vi "Digital_Bridge_3_kart.vi"() -> ()   [LabVIEW 2014] (continued)
                    n5059 = local write "IF ELSE Y 5"(w1698) -> ()
                    n5060 = local write "Y1 2"(w1698) -> ()
                    n5061 = local write "IF ELSE Y"(w1698) -> ()
                    n5062 = local write "X1 3"(w1698) -> ()
                    n5063 = local write "IF ELSE X"(w1698) -> ()
                    n5064 = local write "Y1 3"(w1698) -> ()
                    n5065 = local write "RANGE KONTROL X"(w1698) -> ()
                    n5066 = local write "Y 4"(w1698) -> ()
                    n5067 = local write "RANGE KONTROL Y 2"(w1698) -> ()
                    n5068 = local write "Y"(w1698) -> ()
                    n5069 = local write "RANGE KONTROL Y 3"(w1698) -> ()
                    n5070 = local write "X 5"(w1698) -> ()
                    n5071 = local write "RANGE KONTROL X 4"(w1698) -> ()
                    n5072 = local write "Y 5"(w1698) -> ()
                    n5073 = local write "RANGE KONTROL Y 4"(w1698) -> ()
                    n5074 = local write "IF ELSE Y 2"(w1698) -> ()
                    n5075 = local write "X1 4"(w1698) -> ()
                    n5076 = local write "IF ELSE X 2"(w1698) -> ()
                    n5077 = local write "Y1 4"(w1698) -> ()
                    n5078 = local write "IF ELSE Y 3"(w1698) -> ()
                    n5079 = local write "X1 5"(w1698) -> ()
                    n5080 = local write "IF ELSE X 3"(w1698) -> ()
                    n5081 = local write "Y1 5"(w1698) -> ()
                    n5082 = local write "IF ELSE X 4"(w1698) -> ()
                    "Boolean 5" <- w1696
                    "Boolean 3" <- w1696
                    "Boolean 2" <- w1696
                    "Boolean 4" <- w1696
                    "Boolean" <- w1696
                  }
                }
                n5083 = flat-sequence {
                  frame #0 {
                    w1411 = dbl[][] [] ("Other Array")
                    w1412 = dbl[][] [] ("Other Array")
                    "Denge Kosulu x2_y2" <- w1412
                    "Denge Kosulu x1_x2" <- w1412
                    "Denge Kosulu y1_y2" <- w1412
                    "Output Denge Kosulu x2_y2" <- w1411
                    "Output Denge Kosulu x1_x2" <- w1411
                    "Outpu Denge Kosulu y1_y2" <- w1411
                  }
                  frame #1 {
                    n5084 = Initialize Array(0.0 ("element"), 10 ("dimension size"), 20 ("dimension size")) -> (w1416:dbl[][])
                    n5085 = Initialize Array(0.0 ("element"), 10 ("dimension size"), 20 ("dimension size")) -> (w1417:dbl[][])
                    n5086 = Initialize Array(0.0 ("element"), 10 ("dimension size"), 20 ("dimension size")) -> (w1418:dbl[][])
                    n5087 = local write "Denge Kosulu x2_y2"(w1418) -> ()
                    n5088 = local write "Denge Kosulu y1_y2"(w1416) -> ()
                    n5089 = local write "Denge Kosulu x1_x2"(w1417) -> ()
                  }
                  frame #2 {
                    n5090 = for {
                      N: 20 -> [_]
                      i -> [w1426]
                      n5091 = for {
                        N: 10 -> [_]
                        tunnel: w1426 -> [w1428]
                        i -> [w1431]
                        n5092 = local read "Denge Kosulu x2_y2"() -> (w1430:dbl[][])
                        n5093 = case shown="5" w1431 {
                          tunnel: w1431 -> [w1435 w1439 w1445 w1450 w1455 w1460 w1465 w1470 w1475 w1480]
                          tunnel: w1430 -> [w1434 w1438 w1444 w1449 w1454 w1459 w1464 w1469 w1474 w1479]
                          tunnel: [w1433 w1440 w1443 w1448 w1453 w1458 w1463 w1468 w1473 w1478] -> w1429
                          tunnel: w1428 -> [w1432 w1437 w1442 w1447 w1452 w1457 w1462 w1467 w1472 w1477]
                          frame 0, Default {
                            n5094 = local read "AD X_2"() -> (w1436:dbl)
                            n5095 = Replace Array Subset(array=w1434, new element=w1436, index (row)=w1435, index (col)=w1432) -> (w1433:dbl[][])
                          }
                          frame 1 {
                            n5096 = local read "AD Y_2"() -> (w1441:dbl)
                            n5097 = Replace Array Subset(array=w1438, new element=w1441, index (row)=w1439, index (col)=w1437) -> (w1440:dbl[][])
                          }
                          frame 2 {
                            n5098 = local read "10R X_2"() -> (w1446:dbl)
                            n5099 = Replace Array Subset(array=w1444, new element=w1446, index (row)=w1445, index (col)=w1442) -> (w1443:dbl[][])
                          }
                          frame 3 {
                            n5100 = local read "10R Y_2"() -> (w1451:dbl)
                            n5101 = Replace Array Subset(array=w1449, new element=w1451, index (row)=w1450, index (col)=w1447) -> (w1448:dbl[][])
                          }
                          frame 4 {
                            n5102 = local read "1R X_2"() -> (w1456:dbl)
                            n5103 = Replace Array Subset(array=w1454, new element=w1456, index (row)=w1455, index (col)=w1452) -> (w1453:dbl[][])
                          }
                          frame 5 {
                            n5104 = local read "1R Y_2"() -> (w1461:dbl)
                            n5105 = Replace Array Subset(array=w1459, new element=w1461, index (row)=w1460, index (col)=w1457) -> (w1458:dbl[][])
                          }
                          frame 6 {
                            n5106 = local read "Wagner X_2"() -> (w1466:dbl)
                            n5107 = Replace Array Subset(array=w1464, new element=w1466, index (row)=w1465, index (col)=w1462) -> (w1463:dbl[][])
                          }
                          frame 7 {
                            n5108 = local read "Wagner Y_2"() -> (w1471:dbl)
                            n5109 = Replace Array Subset(array=w1469, new element=w1471, index (row)=w1470, index (col)=w1467) -> (w1468:dbl[][])
                          }
                          frame 8 {
                            n5110 = local read "Kelvin X_2"() -> (w1476:dbl)
                            n5111 = Replace Array Subset(array=w1474, new element=w1476, index (row)=w1475, index (col)=w1472) -> (w1473:dbl[][])
                          }
                          frame 9 {
                            n5112 = local read "Kelvin Y_2"() -> (w1481:dbl)
                            n5113 = Replace Array Subset(array=w1479, new element=w1481, index (row)=w1480, index (col)=w1477) -> (w1478:dbl[][])
                          }
                        }
                        n5114 = local write "Denge Kosulu x2_y2"(w1429) -> ()
                      }
                    }
                  }
                  frame #3 {
                    n5115 = for {
                      N: 20 -> [_]
                      i -> [w1483]
                      n5116 = for {
                        N: 10 -> [_]
                        tunnel: w1483 -> [w1485]
                        i -> [w1488]
                        n5117 = local read "Denge Kosulu x1_x2"() -> (w1487:dbl[][])
                        n5118 = case shown="0, Default" w1488 {
                          tunnel: w1488 -> [w1492 w1496 w1502 w1507 w1512 w1517 w1522 w1527 w1532 w1537]
                          tunnel: w1487 -> [w1491 w1495 w1501 w1506 w1511 w1516 w1521 w1526 w1531 w1536]
                          tunnel: [w1490 w1497 w1500 w1505 w1510 w1515 w1520 w1525 w1530 w1535] -> w1486
                          tunnel: w1485 -> [w1489 w1494 w1499 w1504 w1509 w1514 w1519 w1524 w1529 w1534]
                          frame 0, Default {
                            n5119 = local read "AD X_1"() -> (w1493:dbl)
                            n5120 = Replace Array Subset(array=w1491, new element=w1493, index (row)=w1492, index (col)=w1489) -> (w1490:dbl[][])
                          }
                          frame 1 {
                            n5121 = local read "AD X_2"() -> (w1498:dbl)
                            n5122 = Replace Array Subset(array=w1495, new element=w1498, index (row)=w1496, index (col)=w1494) -> (w1497:dbl[][])
                          }
                          frame 2 {
                            n5123 = local read "10R X_1"() -> (w1503:dbl)
                            n5124 = Replace Array Subset(array=w1501, new element=w1503, index (row)=w1502, index (col)=w1499) -> (w1500:dbl[][])
                          }
                          frame 3 {
                            n5125 = local read "10R X_2"() -> (w1508:dbl)
                            n5126 = Replace Array Subset(array=w1506, new element=w1508, index (row)=w1507, index (col)=w1504) -> (w1505:dbl[][])
                          }
                          frame 4 {
                            n5127 = local read "1R X_1"() -> (w1513:dbl)
                            n5128 = Replace Array Subset(array=w1511, new element=w1513, index (row)=w1512, index (col)=w1509) -> (w1510:dbl[][])
                          }
                          frame 5 {
                            n5129 = local read "1R X_2"() -> (w1518:dbl)
                            n5130 = Replace Array Subset(array=w1516, new element=w1518, index (row)=w1517, index (col)=w1514) -> (w1515:dbl[][])
                          }
                          frame 6 {
                            n5131 = local read "Wagner X_1"() -> (w1523:dbl)
                            n5132 = Replace Array Subset(array=w1521, new element=w1523, index (row)=w1522, index (col)=w1519) -> (w1520:dbl[][])
                          }
                          frame 7 {
                            n5133 = local read "Wagner X_2"() -> (w1528:dbl)
                            n5134 = Replace Array Subset(array=w1526, new element=w1528, index (row)=w1527, index (col)=w1524) -> (w1525:dbl[][])
                          }
                          frame 8 {
                            n5135 = local read "Kelvin X_1"() -> (w1533:dbl)
                            n5136 = Replace Array Subset(array=w1531, new element=w1533, index (row)=w1532, index (col)=w1529) -> (w1530:dbl[][])
                          }
                          frame 9 {
                            n5137 = local read "Kelvin X_2"() -> (w1538:dbl)
                            n5138 = Replace Array Subset(array=w1536, new element=w1538, index (row)=w1537, index (col)=w1534) -> (w1535:dbl[][])
                          }
                        }
                        n5139 = local write "Denge Kosulu x1_x2"(w1486) -> ()
                      }
                    }
                  }
                  frame #4 {
                    n5140 = for {
                      N: 20 -> [_]
                      i -> [w1540]
                      n5141 = for {
                        N: 10 -> [_]
                        tunnel: w1540 -> [w1542]
                        i -> [w1545]
                        n5142 = local read "Denge Kosulu y1_y2"() -> (w1544:dbl[][])
                        n5143 = case shown="8" w1545 {
                          tunnel: w1545 -> [w1549 w1553 w1559 w1564 w1569 w1574 w1579 w1584 w1589 w1594]
                          tunnel: w1544 -> [w1548 w1552 w1558 w1563 w1568 w1573 w1578 w1583 w1588 w1593]
                          tunnel: [w1547 w1554 w1557 w1562 w1567 w1572 w1577 w1582 w1587 w1592] -> w1543
                          tunnel: w1542 -> [w1546 w1551 w1556 w1561 w1566 w1571 w1576 w1581 w1586 w1591]
                          frame 0, Default {
                            n5144 = local read "AD Y_1"() -> (w1550:dbl)
                            n5145 = Replace Array Subset(array=w1548, new element=w1550, index (row)=w1549, index (col)=w1546) -> (w1547:dbl[][])
                          }
                          frame 1 {
                            n5146 = local read "AD Y_2"() -> (w1555:dbl)
                            n5147 = Replace Array Subset(array=w1552, new element=w1555, index (row)=w1553, index (col)=w1551) -> (w1554:dbl[][])
                          }
                          frame 2 {
                            n5148 = local read "10R  Y_1"() -> (w1560:dbl)
                            n5149 = Replace Array Subset(array=w1558, new element=w1560, index (row)=w1559, index (col)=w1556) -> (w1557:dbl[][])
                          }
                          frame 3 {
                            n5150 = local read "10R Y_2"() -> (w1565:dbl)
                            n5151 = Replace Array Subset(array=w1563, new element=w1565, index (row)=w1564, index (col)=w1561) -> (w1562:dbl[][])
                          }
                          frame 4 {
                            n5152 = local read "1R Y_1"() -> (w1570:dbl)
                            n5153 = Replace Array Subset(array=w1568, new element=w1570, index (row)=w1569, index (col)=w1566) -> (w1567:dbl[][])
                          }
                          frame 5 {
                            n5154 = local read "1R Y_2"() -> (w1575:dbl)
                            n5155 = Replace Array Subset(array=w1573, new element=w1575, index (row)=w1574, index (col)=w1571) -> (w1572:dbl[][])
                          }
                          frame 6 {
                            n5156 = local read "Wagner Y_1"() -> (w1580:dbl)
                            n5157 = Replace Array Subset(array=w1578, new element=w1580, index (row)=w1579, index (col)=w1576) -> (w1577:dbl[][])
                          }
                          frame 7 {
                            n5158 = local read "Wagner Y_2"() -> (w1585:dbl)
                            n5159 = Replace Array Subset(array=w1583, new element=w1585, index (row)=w1584, index (col)=w1581) -> (w1582:dbl[][])
                          }
                          frame 8 {
                            n5160 = local read "Kelvin Y_1"() -> (w1590:dbl)
                            n5161 = Replace Array Subset(array=w1588, new element=w1590, index (row)=w1589, index (col)=w1586) -> (w1587:dbl[][])
                          }
                          frame 9 {
                            n5162 = local read "Kelvin Y_2"() -> (w1595:dbl)
                            n5163 = Replace Array Subset(array=w1593, new element=w1595, index (row)=w1594, index (col)=w1591) -> (w1592:dbl[][])
                          }
                        }
                        n5164 = local write "Denge Kosulu y1_y2"(w1543) -> ()
                      }
                    }
                  }
                }
                n5165 = flat-sequence {
                  frame #0 {
                    w1607 = 0.0 ("result output x [Wagner]")
                    w1609 = 0.0 ("output 2 y [10R]")
                    w1610 = 0.0 ("input 2 x [kelvin]")
                    w1611 = 0.0 ("input 1 x [kelvin]")
                    w1614 = 0.0 ("iterasyon ana denge")
                    w1615 = 0.0 ("iterasyon ana denge")
                    w1613 = 0.0 ("input 1 x [10R]")
                    w1612 = 0.0 ("iterasyon ana denge")
                    n5166 = global read "First_input_values.vi" "Active"() -> (w1606:bool)
                    n5167 = case shown="True" w1606 {
                      frame False {
                        n5168 = global read "First_input_values.vi" "Y 2. input 1R"() -> (→"Y 2.input 1R" →"1R Y(k-1)":dbl)
                        n5169 = global read "First_input_values.vi" "Y 1. input 1R"() -> (→"Y 1.input 1R" →"1R Yk":dbl)
                        n5170 = global read "First_input_values.vi" "X 2. input 1R"() -> (→"X 2.input 1R" →"1R X(k-1)":dbl)
                        n5171 = global read "First_input_values.vi" "X 1. input 1R"() -> (→"X 1.input 1R" →"1R Xk":dbl)
                        n5172 = global read "First_input_values.vi" "X 1. input 10R"() -> (→"X 1.input 10R" →"10R Xk":dbl)
                        n5173 = global read "First_input_values.vi" "X 2. input 10R"() -> (→"X 2.input 10R" →"10R X(k-1)":dbl)
                        n5174 = global read "First_input_values.vi" "X 1. input AD"() -> (→"X 1.input AD" →"AD Xk":dbl)
                        n5175 = global read "First_input_values.vi" "X 2. input AD"() -> (→"X 2.input AD" →"AD X(k-1)":dbl)
                        n5176 = global read "First_input_values.vi" "Y 2. input AD"() -> (→"Y 2.input AD" →"AD Y(k-1)":dbl)
                        n5177 = global read "First_input_values.vi" "Y 2. input 10R"() -> (→"Y 2.input 10R" →"10R Y(k-1)":dbl)
                        n5178 = global read "First_input_values.vi" "Y 1. input AD"() -> (→"Y 1.input AD" →"AD Yk":dbl)
                        n5179 = global read "First_input_values.vi" "Y 1. input 10R"() -> (→"Y 1.input 10R" →"10R Yk":dbl)
                        n5180 = global read "First_input_values.vi" "Y 1. input KV"() -> (→"Y 1.input KV" →"Kelvin Yk":dbl)
                        n5181 = global read "First_input_values.vi" "Y 2. input KV"() -> (→"Y 2.input KV" →"Kelvin Y(k-1)":dbl)
                        n5182 = global read "First_input_values.vi" "X 1. input KV"() -> (→"X 1.input KV" →"Kelvin Xk":dbl)
                        n5183 = global read "First_input_values.vi" "X 2. input KV"() -> (→"X 2.input KV" →"Kelvin X(k-1)":dbl)
                        n5184 = global read "First_input_values.vi" "X 2. input W"() -> (→"X 2.input W" →"Wagner  X(k-1)":dbl)
                        n5185 = global read "First_input_values.vi" "X 1. input W"() -> (→"X 1.input W" →"Wagner Xk":dbl)
                        n5186 = global read "First_input_values.vi" "Y 1. input W"() -> (→"Y 1.input W" →"Wagner Yk":dbl)
                        n5187 = global read "First_input_values.vi" "Y 2. input W"() -> (→"Y 2.input W" →"Wagner Y(k-1)":dbl)
                        n5188 = global read "First_input_values.vi" "X range 10R"() -> (→"X Range 10R":dbl)
                        n5189 = global read "First_input_values.vi" "X range AD"() -> (→"X Range AD":dbl)
                        n5190 = global read "First_input_values.vi" "X range KV"() -> (→"X Range KV":dbl)
                        n5191 = global read "First_input_values.vi" "X range 1R"() -> (→"X Range 1R":dbl)
                        n5192 = global read "First_input_values.vi" "X range W"() -> (→"X Range W":dbl)
                        n5193 = global read "First_input_values.vi" "Y range 10R"() -> (→"Y Range 10R":dbl)
                        n5194 = global read "First_input_values.vi" "Y range AD"() -> (→"Y Range AD":dbl)
                        n5195 = global read "First_input_values.vi" "Y range KV"() -> (→"Y Range KV":dbl)
                        n5196 = global read "First_input_values.vi" "Y range 1R"() -> (→"Y Range 1R":dbl)
                        n5197 = global read "First_input_values.vi" "Y range W"() -> (→"Y Range W":dbl)
                      }
                      frame True {
                        n5198 = for {
                          N: 6 -> [_]
                          i -> [w1648]
                          n5199 = for {
                            N: 5 -> [_]
                            tunnel: w1648 -> [w1651]
                            i -> [w1650]
                            n5200 = global read "First_input_values.vi" "Multi Values"() -> (w1653:dbl[][][])
                            n5201 = Index Array(array=w1653, index (dim 0)=0 ("index (page)"), index (dim 1)=w1651, index (dim 2)=w1650) -> (element=w1649:dbl)
                            n5202 = case shown="0, Default" w1651 {
                              tunnel: w1650 -> [w1655 w1662 w1669 w1676 w1683 w1690]
                              tunnel: w1649 -> [w1654 w1661 w1668 w1675 w1682 w1689]
                              frame 0, Default {
                                n5203 = case shown="0, Default" w1655 {
                                tunnel: w1654 -> [w1656 w1657 w1658 w1659 w1660]
                                frame 0, Default {
                                n5204 = local write "AD Xk"(w1656) -> ()
                                n5205 = local write "X 1.input AD"(w1656) -> ()
                                }
                                frame 1 {
                                n5206 = local write "10R Xk"(w1657) -> ()
                                n5207 = local write "X 1.input 10R"(w1657) -> ()
                                }
                                frame 2 {
                                n5208 = local write "1R Xk"(w1658) -> ()
                                n5209 = local write "X 1.input 1R"(w1658) -> ()
                                }
                                frame 3 {
                                n5210 = local write "Wagner Xk"(w1659) -> ()
                                n5211 = local write "X 1.input W"(w1659) -> ()
                                }
                                frame 4 {
                                n5212 = local write "Kelvin Xk"(w1660) -> ()
                                n5213 = local write "X 1.input KV"(w1660) -> ()
                                }
                                }
                              }
                              frame 1 {
                                n5214 = case shown="0, Default" w1662 {
                                tunnel: w1661 -> [w1663 w1664 w1665 w1666 w1667]
                                frame 0, Default {
                                n5215 = local write "AD X(k-1)"(w1663) -> ()
                                n5216 = local write "X 2.input AD"(w1663) -> ()
                                }
                                frame 1 {
                                n5217 = local write "10R X(k-1)"(w1664) -> ()
                                n5218 = local write "X 2.input 10R"(w1664) -> ()
                                }
                                frame 2 {
                                n5219 = local write "1R X(k-1)"(w1665) -> ()
                                n5220 = local write "X 2.input 1R"(w1665) -> ()
                                }
                                frame 3 {
                                n5221 = local write "Wagner  X(k-1)"(w1666) -> ()
                                n5222 = local write "X 2.input W"(w1666) -> ()
                                }
                                frame 4 {
                                n5223 = local write "Kelvin X(k-1)"(w1667) -> ()
                                n5224 = local write "X 2.input KV"(w1667) -> ()
                                }
                                }
                              }
                              frame 2 {
                                n5225 = case shown="2" w1669 {
                                tunnel: w1668 -> [w1670 w1671 w1672 w1673 w1674]
                                frame 0, Default {
                                n5226 = local write "X Range AD"(w1670) -> ()
                                }
                                frame 1 {
                                n5227 = local write "X Range 10R"(w1671) -> ()
                                }
                                frame 2 {
                                n5228 = local write "X Range 1R"(w1672) -> ()
                                }
                                frame 3 {
                                n5229 = local write "X Range W"(w1673) -> ()
                                }
                                frame 4 {
                                n5230 = local write "X Range KV"(w1674) -> ()
                                }
                                }
                              }
                              frame 3 {
                                n5231 = case shown="0, Default" w1676 {
                                tunnel: w1675 -> [w1677 w1678 w1679 w1680 w1681]
                                frame 0, Default {
                                n5232 = local write "AD Yk"(w1677) -> ()
                                n5233 = local write "Y 1.input AD"(w1677) -> ()
                                }
                                frame 1 {
                                n5234 = local write "10R Yk"(w1678) -> ()
                                n5235 = local write "Y 1.input 10R"(w1678) -> ()
                                }
                                frame 2 {
                                n5236 = local write "1R Yk"(w1679) -> ()
                                n5237 = local write "Y 1.input 1R"(w1679) -> ()
                                }
                                frame 3 {
                                n5238 = local write "Wagner Yk"(w1680) -> ()
                                n5239 = local write "Y 1.input W"(w1680) -> ()
                                }
                                frame 4 {
                                n5240 = local write "Kelvin Yk"(w1681) -> ()
                                n5241 = local write "Y 1.input KV"(w1681) -> ()
                                }
                                }
                              }
                              frame 4 {
                                n5242 = case shown="0, Default" w1683 {
                                tunnel: w1682 -> [w1684 w1685 w1686 w1687 w1688]
                                frame 0, Default {
                                n5243 = local write "AD Y(k-1)"(w1684) -> ()
                                n5244 = local write "Y 2.input AD"(w1684) -> ()
                                }
                                frame 1 {
                                n5245 = local write "10R Y(k-1)"(w1685) -> ()
                                n5246 = local write "Y 2.input 10R"(w1685) -> ()
                                }
                                frame 2 {
                                n5247 = local write "1R Y(k-1)"(w1686) -> ()
                                n5248 = local write "Y 2.input 1R"(w1686) -> ()
                                }
                                frame 3 {
                                n5249 = local write "Wagner Y(k-1)"(w1687) -> ()
                                n5250 = local write "Y 2.input W"(w1687) -> ()
                                }
                                frame 4 {
                                n5251 = local write "Kelvin Y(k-1)"(w1688) -> ()
                                n5252 = local write "Y 2.input KV"(w1688) -> ()
                                }
                                }
                              }
                              frame 5 {
                                n5253 = case shown="0, Default" w1690 {
                                tunnel: w1689 -> [w1691 w1692 w1693 w1694 w1695]
                                frame 0, Default {
                                n5254 = local write "Y Range AD"(w1691) -> ()
                                }
                                frame 1 {
                                n5255 = local write "Y Range 10R"(w1692) -> ()
                                }
                                frame 2 {
                                n5256 = local write "Y Range 1R"(w1693) -> ()
                                }
                                frame 3 {
                                n5257 = local write "Y Range W"(w1694) -> ()
                                }
                                frame 4 {
                                n5258 = local write "Y Range KV"(w1695) -> ()
                                }
                                }
                              }
                            }
                          }
                        }
                      }
                    }
                    "input 1 x [kelvin]" <- w1610
                    "input 2 x [kelvin]" <- w1610
                    "output 2 x [kelvin]" <- w1610
                    "output 1 x [kelvin]" <- w1610
                    "input 1 y [kelvin]" <- w1610
                    "input 2 y [kelvin]" <- w1610
                    "output 1 y [kelvin]" <- w1610
                    "output 2 y [kelvin]" <- w1610
                    "input 1 x [wagner]" <- w1611
                    "input 2 x [wagner]" <- w1611
                    "output 1 x [wagner]" <- w1611
                    "output 2 x [wagner]" <- w1611
                    "input 1 y [wagner]" <- w1611
                    "input 2 y [wagner]" <- w1611
                    "output 1 y [wagner]" <- w1611
                    "output 2 y [wagner]" <- w1611
                    "output 2 x [1R]" <- w1612
                    "output 1 x [1R]" <- w1612
                    "input 1 x [1R]" <- w1612
                    "input 2 x [1R]" <- w1612
                    "input 1 y [1R]" <- w1612
                    "input 2 y [1R]" <- w1612
                    "output 1 y [1R]" <- w1612
                    "output 2 y [1R]" <- w1612
                    "output 1 x [10R]" <- w1609
                    "input 1 x [10R]" <- w1609
                    "output 2 x [10R]" <- w1609
                    "input 2 x [10R]" <- w1609
                    "input 2 y [10R]" <- w1609
                    "output 2 y [10R]" <- w1609
                    "input 1 y [10R]" <- w1609
                    "output 1 y [10R]" <- w1609
                    "output 2 x [ana denge]" <- w1613
                    "output 1 x [ana denge]" <- w1613
                    "input 1 x [ana denge]" <- w1613
                    "input 2 x [ana denge]" <- w1613
                    "input 1 y [ana denge]" <- w1613
                    "input 2 y [ana denge]" <- w1613
                    "output 2 y [ana denge]" <- w1613
                    "output 1 y [ana denge]" <- w1613
                    "iterasyon KELVIN" <- w1615
                    "iterasyon WAGNER" <- w1615
                    "iterasyon 1R" <- w1615
                    "iterasyon 10R" <- w1615
                    "iterasyon AD" <- w1615
                    "İterasyon X" <- w1614
                    "İterasyon Y" <- w1614
                    "İterasyon X 2" <- w1614
                    "İterasyon Y 2" <- w1614
                    "İterasyon X 3" <- w1614
                    "İterasyon Y 3" <- w1614
                    "İterasyon X 4" <- w1614
                    "İterasyon Y 4" <- w1614
                    "İterasyon X 5" <- w1614
                    "İterasyon Y 5" <- w1614
                    "Iterasyon Successful" <- 0.0 ("Iterasyon Successful")
                    "result output x [Wagner]" <- w1607
                    "result output y [Wagner]" <- w1607
                    "result output x [1R]" <- w1607
                    "result output y [1R]" <- w1607
                    "result output x [10R]" <- w1607
                    "result output y [10R]" <- w1607
                    "result output x [AD]" <- w1607
                    "result output y [AD]" <- w1607
                    "result output x [Kelvin]" <- w1607
                    "result output y [Kelvin]" <- w1607
                  }
                }
                n5259 = flat-sequence {
                  frame #0 {
                    "Hatalar" <- string[] [] ("Hatalar")
                    "Frekanslar" <- i32[] []
                    "extra default values" <- i32[][] []
                    "control hz array" <- i32[][] []
                  }
                }
                n5260 = flat-sequence {
                  tunnel: [w1596] -> w1410
                  tunnel: w1410 -> [w1598]
                  frame #0 {
                    n5261 = property on="Frekans Listbox" class="LstBox (strict)"() -> ("Item Names"=w1596:string[])  [unwired: 2 in, 2 out]
                    n5262 = property on="Multicolumn Listbox" class="MCListbox (strict)"("RowHdrs[]"=w1596) -> ()  [unwired: 2 in, 2 out]
                  }
                  frame #1 {
                    n5263 = Array Size(array=w1598) -> (size(s)=w1597:i32)
                    n5264 = property on="Multicolumn Listbox" class="MCListbox (strict)"("NumRows"=w1597) -> ()  [unwired: 2 in, 2 out]
                  }
                  frame #2 {
                    n5265 = property on="Frekans Listbox" class="LstBox (strict)"() -> ("Item Names"=w1599:string[])  [unwired: 2 in, 2 out]
                    n5266 = Array Size(array=w1599) -> (size(s)=w1600:i32)
                    n5267 = for {
                      N: w1600 -> [_]
                      i -> [w1604]
                      n5268 = property on="Multicolumn Listbox" class="MCListbox (strict)"() -> ("RowHdrs[]"=w1602:string[])  [unwired: 2 in, 2 out]
                      n5269 = property on="Frekans Listbox" class="LstBox (strict)"() -> ("Item Names"=w1605:string[])  [unwired: 2 in, 2 out]
                      n5270 = Index Array(array=w1605, index=w1604) -> (element=w1603:string)
                      n5271 = Replace Array Subset(array=w1602, new element=w1603, index=w1604) -> (w1601:string[])
                      n5272 = property on="Multicolumn Listbox" class="MCListbox (strict)"("RowHdrs[]"=w1601) -> ()  [unwired: 2 in, 2 out]
                    }
                  }
                }
              }
              frame #1 {
                n5273 = local write "first process"(FALSE ("first process")) -> ()
              }
            }
          }
        }
        n5274 = case shown="True" "error" {
          frame False {
          }
          frame True {
            n5275 = disable-structure shown="Disabled" {
              frame Disabled {
                n5276 = local read "Denge Seçimi"() -> (w1765:u8)
                n5277 = Number To Fractional String(number=w1765) -> ()  [unwired: 3 in, 1 out]
              }
              frame Enabled {
              }
            }
            n5278 = local read "frekans index"() -> (w1762:dbl)
            n5279 = local read "Frekanslar"() -> (w1763:dbl[])
            n5280 = Index Array(array=w1763, index=w1762) -> (element=w1764:dbl)
            n5281 = Number To Decimal String(number=w1764) -> (decimal integer string=w1759:string)  [unwired: 1 in]
            n5282 = Concatenate Strings(w1759, " Hz dengelenemedi") -> (w1757:string)
            n5283 = flat-sequence {
              tunnel: [w1766] -> w1761
              tunnel: w1757 -> [w1766]
              tunnel: [w1768] -> w1760
              tunnel: w1761 -> [w1768]
              tunnel: w1760 -> [w1770]
              frame #0 {
                n5284 = Wait (ms)(milliseconds to wait=u32 1000) -> ()  [unwired: 1 out]
              }
              frame #1 {
                n5285 = disable-structure shown="Disabled" {
                  frame Disabled {
                    w1769 = "a" ("button name (\"OK\")")
                    n5286 = One Button Dialog(message=w1769, button name ("OK")=w1769) -> ()  [unwired: 1 out]
                  }
                  frame Enabled {
                  }
                }
              }
              frame #2 {
                n5287 = flat-sequence {
                  tunnel: w1770 -> [w1776]
                  tunnel: [w1774] -> w1773
                  tunnel: [w1777] -> w1772
                  tunnel: w1773 -> [w1777]
                  tunnel: [w1779] -> w1771
                  tunnel: w1772 -> [w1779]
                  tunnel: w1771 -> [w1781]
                  frame #0 {
                    n5288 = local read "Hatalar"() -> (w1775:string[])
                    n5289 = Build Array (concatenate)(w1776, w1775) -> (w1774:string[])
                  }
                  frame #1 {
                    n5290 = local write "Hatalar"(string[] [] ("Hatalar")) -> ()
                  }
                  frame #2 {
                    n5291 = Wait (ms)(milliseconds to wait=u32 100) -> ()  [unwired: 1 out]
                  }
                  frame #3 {
                    n5292 = local write "Hatalar"(w1781) -> ()
                  }
                }
              }
              frame #3 {
                n5293 = local write "reset values"(TRUE ("reset values")) -> ()
                n5294 = local write "error 2"(TRUE ("reset values")) -> ()
                n5295 = local write "error"(FALSE ("reset values")) -> ()
              }
            }
            n5296 = local read "input values"() -> (→"input values 2":dbl[])
          }
        }
        n5297 = case shown="True" "Wagner" {
          frame False {
          }
          frame True {
            n5298 = flat-sequence {
              frame #0 {
                w674 = u16 0 items=["Wagner", "Ground"] ("Switch")
                w673 = u16 1 items=["Open All", "Ana Denge", "10R", "1R"] ("Ring")
                n5299 = call "mux1.vi"("Ring"=w673) -> ("error out"=w672:errorcluster)  [unwired: 9 in]
                n5300 = call "mux2.vi"("Switch"=w674, "error in (no error)"=w672) -> ()  [unwired: 6 in, 1 out]
              }
              frame #1 {
                n5301 = Wait (ms)(milliseconds to wait=u32 100) -> ()  [unwired: 1 out]
              }
              frame #2 {
                w677 = u16 0 items=["A", "A-B"] ("Input Source (0: A)")
                n5302 = local read "GPIB In"() -> (w676:refnum<visa-resource-name>)
                n5303 = call "input source.vi"("Input Source (0: A)"=w677, "VISA resource name"=w676) -> ()  [unwired: 8 in, 2 out]
              }
              frame #3 {
                n5304 = Wait (ms)(milliseconds to wait=u32 100) -> ()  [unwired: 1 out]
              }
              frame #4 {
                n5305 = local write "Wagner"(FALSE) -> ()
              }
            }
          }
        }
        n5306 = case shown="True" "Kelvin" {
          frame False {
          }
          frame True {
            n5307 = flat-sequence {
              frame #0 {
                w666 = u16 1 items=["Wagner", "Ground"] ("Switch")
                w665 = u16 1 items=["Open All", "Ana Denge", "10R", "1R"] ("Ring")
                n5308 = call "mux1.vi"("Ring"=w665) -> ("error out"=w664:errorcluster)  [unwired: 9 in]
                n5309 = call "mux2.vi"("Switch"=w666, "error in (no error)"=w664) -> ()  [unwired: 6 in, 1 out]
              }
              frame #1 {
                n5310 = Wait (ms)(milliseconds to wait=u32 100) -> ()  [unwired: 1 out]
              }
              frame #2 {
                w669 = u16 1 items=["A", "A-B"] ("Input Source (0: A)")
                n5311 = local read "GPIB In"() -> (w668:refnum<visa-resource-name>)
                n5312 = call "input source.vi"("Input Source (0: A)"=w669, "VISA resource name"=w668) -> ()  [unwired: 8 in, 2 out]
              }
              frame #3 {
                n5313 = Wait (ms)(milliseconds to wait=u32 100) -> ()  [unwired: 1 out]
              }
              frame #4 {
                n5314 = local write "Kelvin"(FALSE) -> ()
              }
            }
          }
        }
        n5315 = case shown="True" "Open all" {
          frame False {
          }
          frame True {
            n5316 = flat-sequence {
              frame #0 {
                w658 = u16 1 items=["Wagner", "Ground"] ("Switch")
                w657 = u16 0 items=["Open All", "Ana Denge", "10R", "1R"] ("Ring")
                n5317 = call "mux1.vi"("Ring"=w657) -> ("error out"=w656:errorcluster)  [unwired: 9 in]
                n5318 = call "mux2.vi"("Switch"=w658, "error in (no error)"=w656) -> ()  [unwired: 6 in, 1 out]
              }
              frame #1 {
                n5319 = Wait (ms)(milliseconds to wait=u32 100) -> ()  [unwired: 1 out]
              }
              frame #2 {
                w661 = u16 0 items=["A", "A-B"] ("Input Source (0: A)")
                n5320 = local read "GPIB In"() -> (w660:refnum<visa-resource-name>)
                n5321 = call "input source.vi"("Input Source (0: A)"=w661, "VISA resource name"=w660) -> ()  [unwired: 8 in, 2 out]
              }
              frame #3 {
                n5322 = Wait (ms)(milliseconds to wait=u32 100) -> ()  [unwired: 1 out]
              }
              frame #4 {
                n5323 = local write "Open all"(FALSE) -> ()
              }
            }
          }
        }
        n5324 = case shown="True" "AD" {
          frame False {
          }
          frame True {
            n5325 = flat-sequence {
              frame #0 {
                w698 = u16 1 items=["Wagner", "Ground"] ("Switch")
                w697 = u16 1 items=["Open All", "Ana Denge", "10R", "1R"] ("Ring")
                n5326 = call "mux1.vi"("Ring"=w697) -> ("error out"=w696:errorcluster)  [unwired: 9 in]
                n5327 = call "mux2.vi"("Switch"=w698, "error in (no error)"=w696) -> ()  [unwired: 6 in, 1 out]
              }
              frame #1 {
                n5328 = Wait (ms)(milliseconds to wait=u32 100) -> ()  [unwired: 1 out]
              }
              frame #2 {
                w701 = u16 0 items=["A", "A-B"] ("Input Source (0: A)")
                n5329 = local read "GPIB In"() -> (w700:refnum<visa-resource-name>)
                n5330 = call "input source.vi"("Input Source (0: A)"=w701, "VISA resource name"=w700) -> ()  [unwired: 8 in, 2 out]
              }
              frame #3 {
                n5331 = Wait (ms)(milliseconds to wait=u32 100) -> ()  [unwired: 1 out]
              }
              frame #4 {
                n5332 = local write "AD"(FALSE) -> ()
              }
            }
          }
        }
        n5333 = case shown="True" "1R" {
          frame False {
          }
          frame True {
            n5334 = flat-sequence {
              frame #0 {
                w682 = u16 1 items=["Wagner", "Ground"] ("Switch")
                w681 = u16 3 items=["Open All", "Ana Denge", "10R", "1R"] ("Ring")
                n5335 = call "mux1.vi"("Ring"=w681) -> ("error out"=w680:errorcluster)  [unwired: 9 in]
                n5336 = call "mux2.vi"("Switch"=w682, "error in (no error)"=w680) -> ()  [unwired: 6 in, 1 out]
              }
              frame #1 {
                n5337 = Wait (ms)(milliseconds to wait=u32 100) -> ()  [unwired: 1 out]
              }
              frame #2 {
                w685 = u16 0 items=["A", "A-B"] ("Input Source (0: A)")
                n5338 = local read "GPIB In"() -> (w684:refnum<visa-resource-name>)
                n5339 = call "input source.vi"("Input Source (0: A)"=w685, "VISA resource name"=w684) -> ()  [unwired: 8 in, 2 out]
              }
              frame #3 {
                n5340 = Wait (ms)(milliseconds to wait=u32 100) -> ()  [unwired: 1 out]
              }
              frame #4 {
                n5341 = local write "1R"(FALSE) -> ()
              }
            }
          }
        }
        n5342 = case shown="True" "10R" {
          frame False {
          }
          frame True {
            n5343 = flat-sequence {
              frame #0 {
                w690 = u16 1 items=["Wagner", "Ground"] ("Switch")
                w689 = u16 2 items=["Open All", "Ana Denge", "10R", "1R"] ("Ring")
                n5344 = call "mux1.vi"("Ring"=w689) -> ("error out"=w688:errorcluster)  [unwired: 9 in]
                n5345 = call "mux2.vi"("Switch"=w690, "error in (no error)"=w688) -> ()  [unwired: 6 in, 1 out]
              }
              frame #1 {
                n5346 = Wait (ms)(milliseconds to wait=u32 100) -> ()  [unwired: 1 out]
              }
              frame #2 {
                w693 = u16 0 items=["A", "A-B"] ("Input Source (0: A)")
                n5347 = local read "GPIB In"() -> (w692:refnum<visa-resource-name>)
                n5348 = call "input source.vi"("Input Source (0: A)"=w693, "VISA resource name"=w692) -> ()  [unwired: 8 in, 2 out]
              }
              frame #3 {
                n5349 = Wait (ms)(milliseconds to wait=u32 100) -> ()  [unwired: 1 out]
              }
              frame #4 {
                n5350 = local write "10R"(FALSE) -> ()
              }
            }
          }
        }
        n5351 = call "Role_Auto_Secim.vi"("Activate"="Activate", "Denge Kolu"="Denge Kolu") -> ()  [unwired: 10 in]
        n5352 = case shown="True" "REFERANS FAZ" {
          frame False {
          }
          frame True {
            n5353 = flat-sequence {
              frame #0 {
                n5354 = local read "GPIB In"() -> (w4267:refnum<visa-resource-name>)
                n5355 = call "reference phase.vi"("Reference Phase (0.000 degrees)"="Reference Phase (0.000 degrees)", "VISA resource name"=w4267) -> ()  [unwired: 8 in, 2 out]
              }
              frame #1 {
                n5356 = Wait (ms)(milliseconds to wait=u32 100) -> ()  [unwired: 1 out]
              }
              frame #2 {
                n5357 = local write "REFERANS FAZ"(FALSE ("REFERANS FAZ")) -> ()
              }
            }
          }
        }
        n5358 = case shown="True" "INPUT SOURCE" {
          frame False {
          }
          frame True {
            n5359 = flat-sequence {
              frame #0 {
                n5360 = local read "GPIB In"() -> (w4263:refnum<visa-resource-name>)
                n5361 = call "input source.vi"("Input Source (0: A)"="Input Source (0: A)", "VISA resource name"=w4263) -> ()  [unwired: 8 in, 2 out]
              }
              frame #1 {
                n5362 = Wait (ms)(milliseconds to wait=u32 100) -> ()  [unwired: 1 out]
              }
              frame #2 {
                n5363 = local write "INPUT SOURCE"(FALSE ("REFERANS FAZ")) -> ()
              }
            }
          }
        }
        n5364 = case shown="True" "SENSITIVITY" {
          frame False {
          }
          frame True {
            n5365 = flat-sequence {
              frame #0 {
                n5366 = local read "GPIB In"() -> (w4259:refnum<visa-resource-name>)
                n5367 = call "sensitivity_.vi"("Sensitivity In"="Sensitivity", "VISA resource name"=w4259) -> ()  [unwired: 8 in, 2 out]
              }
              frame #1 {
                n5368 = Wait (ms)(milliseconds to wait=u32 100) -> ()  [unwired: 1 out]
              }
              frame #2 {
                n5369 = local write "SENSITIVITY"(FALSE ("REFERANS FAZ")) -> ()
              }
            }
          }
        }
        n5370 = case shown="True" "SWITCH" {
          frame False {
          }
          frame True {
            n5371 = call "mux1.vi"("Ring"="Mux1") -> ("error out"=w4257:errorcluster)  [unwired: 9 in]
            n5372 = call "mux2.vi"("Switch"="Mux2", "error in (no error)"=w4257) -> ()  [unwired: 6 in, 1 out]
          }
        }
      }
      n5373 = disable-structure shown="Disabled" {
        disable-tunnel: w33 -> [w454 _]
        disable-tunnel: w32 -> [w453 _]
        disable-tunnel: [w452 _] -> w31
        frame Disabled {
          n5374 = call <vilib>:"DAQmx Stop Task.vi"("task/channels in"=w454, "error in"=w453) -> ("task out"=w455:refnum<k21>, "error out"=w456:errorcluster)  [unwired: 12 in]
          n5375 = call <vilib>:"DAQmx Clear Task.vi"("task in"=w455, "error in"=w456) -> ("error out"=w452:errorcluster)  [unwired: 13 in]
        }
        frame Enabled {
        }
      }
      n5376 = disable-structure shown="Disabled" {
        disable-tunnel: w36 -> [w506 _]
        disable-tunnel: w35 -> [w505 _]
        disable-tunnel: [w504 _] -> w34
        frame Disabled {
          n5377 = call <vilib>:"DAQmx Stop Task.vi"("task/channels in"=w506, "error in"=w505) -> ("task out"=w507:refnum<k21>, "error out"=w508:errorcluster)  [unwired: 12 in]
          n5378 = call <vilib>:"DAQmx Clear Task.vi"("task in"=w507, "error in"=w508) -> ("error out"=w504:errorcluster)  [unwired: 13 in]
        }
        frame Enabled {
        }
      }
      n5379 = call <vilib>:"DAQmx Stop Task.vi"("task/channels in"=w204, "error in"=w203) -> ("task out"=w202:refnum<k21>, "error out"=w201:errorcluster)  [unwired: 12 in]
      n5380 = call <vilib>:"DAQmx Stop Task.vi"("task/channels in"=w332, "error in"=w331) -> ("task out"=w334:refnum<k21>, "error out"=w333:errorcluster)  [unwired: 12 in]
      n5381 = call <vilib>:"DAQmx Stop Task.vi"("task/channels in"=w132, "error in"=w133) -> ("task out"=w134:refnum<k21>, "error out"=w135:errorcluster)  [unwired: 12 in]
      n5382 = call <vilib>:"DAQmx Stop Task.vi"("task/channels in"=w345, "error in"=w344) -> ("task out"=w342:refnum<k21>, "error out"=w343:errorcluster)  [unwired: 12 in]
      n5383 = call <vilib>:"DAQmx Stop Task.vi"("task/channels in"=w341, "error in"=w340) -> ("task out"=w338:refnum<k21>, "error out"=w339:errorcluster)  [unwired: 12 in]
      n5384 = call <vilib>:"DAQmx Stop Task.vi"("task/channels in"=w127, "error in"=w126) -> ("task out"=w129:refnum<k21>, "error out"=w128:errorcluster)  [unwired: 12 in]
      n5385 = call <vilib>:"DAQmx Clear Task.vi"("task in"=w334, "error in"=w333) -> ("error out"=w330:errorcluster)  [unwired: 13 in]
      n5386 = call <vilib>:"DAQmx Clear Task.vi"("task in"=w342, "error in"=w343) -> ("error out"=w337:errorcluster)  [unwired: 13 in]
      n5387 = call <vilib>:"DAQmx Clear Task.vi"("task in"=w338, "error in"=w339) -> ("error out"=w336:errorcluster)  [unwired: 13 in]
      n5388 = call <vilib>:"DAQmx Clear Task.vi"("task in"=w202, "error in"=w201) -> ("error out"=w200:errorcluster)  [unwired: 13 in]
      n5389 = call <vilib>:"DAQmx Clear Task.vi"("task in"=w134, "error in"=w135) -> ("error out"=w125:errorcluster)  [unwired: 13 in]
      n5390 = call <vilib>:"DAQmx Clear Task.vi"("task in"=w129, "error in"=w128) -> ("error out"=w124:errorcluster)  [unwired: 13 in]
      n5391 = Merge Errors(w124, w125, w200, w34, w337, w336, w330, w31) -> (w30:errorcluster)
      n5392 = call <vilib>:"Simple Error Handler.vi"("type of dialog (OK msg:1)"=w29, "error in (no error)"=w30) -> ()  [unwired: 3 in, 5 out]
    }
  }
